vi "FTW-Client-Destroy.vi"(0 "FTW-Client In":refnum<class "FTW-Client.lvclass">, 11 "error in":errorcluster) -> (15 "error out":errorcluster)   [LabVIEW 2013, in "FTW-Client.lvclass"]
uses:
  FTW-Client.lvclass
  FTW-Client.lvclass/FTW-Client.ctl
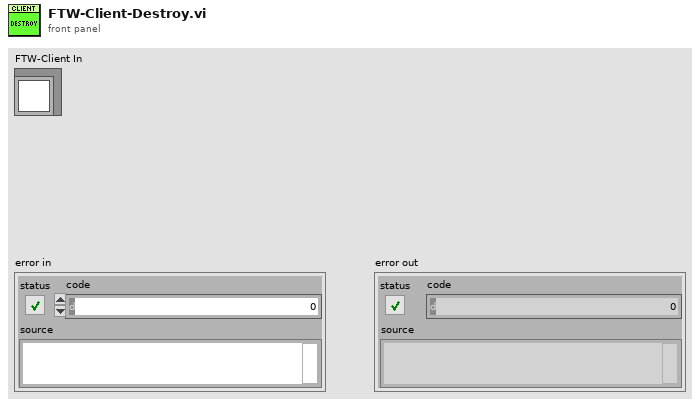
[diagram p1: front panel]
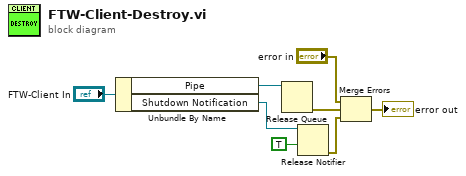
[diagram p0: block diagram]
diagram:
  n1 = Unbundle By Name("FTW-Client In") -> ("Pipe"=w2:refnum<queue>, "Shutdown Notification"=w5:refnum<notifier>)
  n2 = Release Queue(queue=w2) -> (error out=w1:errorcluster)  [unwired: 2 in, 2 out]
  n3 = Release Notifier(notifier=w5, force destroy? (F)=TRUE) -> (error out=w3:errorcluster)  [unwired: 1 in, 2 out]
  n4 = Merge Errors("error in", w1, w3) -> (→"error out":errorcluster)
